vi "Read Columns.vi"(8 "error in (no error)":errorcluster, 11 "DataTable in":refnum<class "DataTable.lvclass">) -> (0 "error out":errorcluster, 2 "Columns":refnum<class "GridColumn.lvclass">[](array[class]), 3 "DataTable out":refnum<class "DataTable.lvclass">)   [LabVIEW 2013, in "DataGrid.lvlib" / "DataTable.lvclass"]
uses:
  DataTable.lvclass
  GridColumn/GridColumn.lvclass
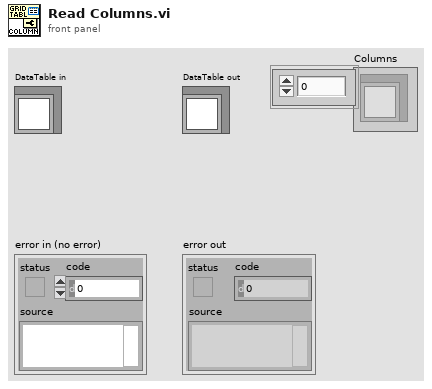
[diagram p1: front panel]
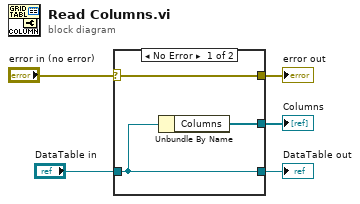
[diagram p0: block diagram]
diagram:
  n1 = case shown="No Error" "error in (no error)" {
    selector: "error in (no error)" -> [w8 w10]
    tunnel: [w8 w10] -> w4
    tunnel: "DataTable in" -> [w7 w9]
    tunnel: [w7 w9] -> w2
    tunnel: [w6 _] -> w1
    frame No Error {
      n2 = Unbundle By Name(w7) -> ("Columns"=w6:refnum<class "GridColumn.lvclass">[])
    }
    frame Error {
    }
  }
  "DataTable out" <- w2
  "error out" <- w4
  "Columns" <- w1
